vi "Search Char.vi"(2 "Search Char":string, 3 "Multiline String":string) -> (0 "Indexes of Char Found":i32[](array[numeric]), 1 "Number of Char Found":i32)   [LabVIEW 2019]
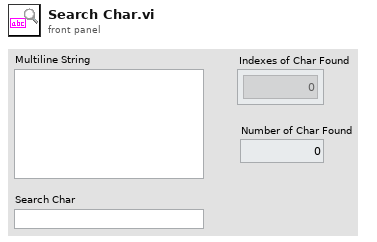
[diagram p1: front panel]
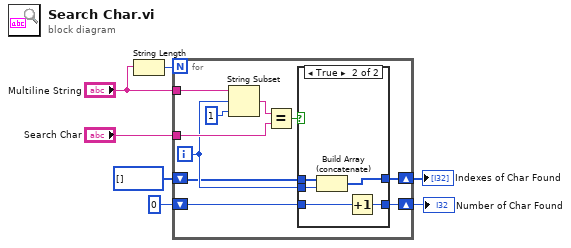
[diagram p0: block diagram]
diagram:
  n1 = String Length(string="Multiline String") -> (length=w6:i32)
  n2 = for {
    N: w6 -> [_]
    tunnel: "Multiline String" -> [w17]
    tunnel: "Search Char" -> [w14]
    shift-right: [w10] -> w2
    shift-left: i32[] [] -> [w11]
    shift-right: [w8] -> w1
    shift-left: 0 -> [w9]
    i -> [w12]
    n3 = String Subset(string=w17, offset (0)=w12, length (rest)=1 ("length (rest)")) -> (substring=w15:string)
    n4 = Equal?(x=w15, y=w14) -> (x = y?=w13:bool)
    n5 = case shown="True" w13 {
      tunnel: w12 -> [_ w24]
      tunnel: w11 -> [w19 w23]
      tunnel: [w19 w22] -> w10
      tunnel: w9 -> [w18 w21]
      tunnel: [w18 w20] -> w8
      frame False {
      }
      frame True {
        n6 = Build Array (concatenate)(w23, w24) -> (w22:i32[])
        n7 = Increment(x=w21) -> (x+1=w20:i32)
      }
    }
  }
  "Indexes of Char Found" <- w2
  "Number of Char Found" <- w1
